vi "LAVA.Parse drawing operation.vi"(6 "picture size":u32, 9 "offset":i32, 11 "picture data in":string) -> (0 "offset past element":i32, 1 "data string":string, 2 "data length":u32, 3 "picture data out":string, 4 "last element":bool, 5 "op-code":T1 items=["set pixel"=4, "move pen"=5, "move pen to"=6, "draw line"=7, "draw line to"=8, "rectangle frame"=9, "rectangle fill"=10, "oval frame"=11, "oval fill"=12, "arc frame"=13, "arc fill"=14, "gray out rect"=15, "poly line"=16, "poly line fill"=17, "text box"=18, "round rect frame"=24, "round rect fill"=25, "copy pixmap"=29, "new font"=0, "copy pixmap with mask"=40, "select pen"=41])   [LabVIEW 2021, in "Pop-Up.lvlib" / "Popup.lvclass"]
doc: "Adapted from : https://lavag.org/topic/17138-2d-picture-translation-movement/#comment-105597"
uses:
  Popup.lvclass
  LAVA.picture op-code.ctl
  Popup.lvclass/Popup.ctl
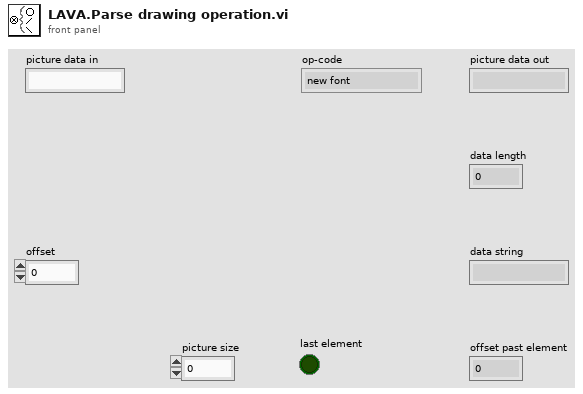
[diagram p1: front panel]
types:
  T1 = typedef "Pop-Up.lvlib/Popup.lvclass/LAVA.picture op-code.ctl" = u16
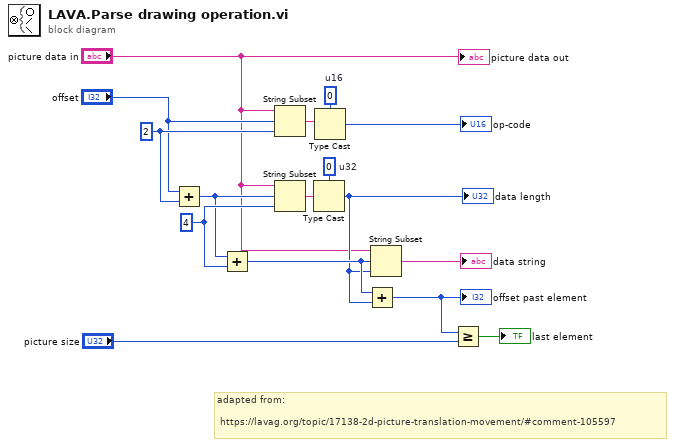
[diagram p0: block diagram]
diagram:
  w12 = u32 0  # u32
  w15 = 4 ("length (rest)")
  w7 = u16 0  # u16
  w11 = 2 ("length (rest)")
  # "adapted from:\n\n https://lavag.org/topic/17138-2d-picture-translation-movement/#comment-105597"
  n1 = Add(x="offset", y=w11) -> (x+y=w14:i32)
  n2 = Add(x=w14, y=w15) -> (x+y=w6:i32)
  n3 = String Subset(string="picture data in", offset (0)="offset", length (rest)=w11) -> (substring=w8:string)
  n4 = String Subset(string="picture data in", offset (0)=w14, length (rest)=w15) -> (substring=w13:string)
  n5 = Type Cast(type=w12, x=w13) -> (*(type *) &x=w5:u32)
  "data length" <- w5
  n6 = Type Cast(type=w7, x=w8) -> (*(type *) &x=→"op-code":u16)
  n7 = Add(x=w6, y=w5) -> (x+y=w3:u32)
  "offset past element" <- w3
  n8 = String Subset(string="picture data in", offset (0)=w6, length (rest)=w5) -> (substring=→"data string":string)
  n9 = Greater Or Equal?(x=w3, y="picture size") -> (x >= y?=→"last element":bool)
  "picture data out" <- "picture data in"
